vi "GetContainedPathSet.vi"(8 "error in (no error)":errorcluster, 11 "CLabVIEWContainer in":refnum<class "CLabVIEWContainer.lvclass">) -> (0 "error out":errorcluster, 1 "Contained":set{string}(c389), 3 "CLabVIEWContainer out":refnum<class "CLabVIEWContainer.lvclass">)   [LabVIEW 2020, in "LabVIEWContainers.lvlib" / "CLabVIEWContainer.lvclass"]
uses:
  CLabVIEWContainer.lvclass
  CLabVIEWContainer.lvclass/CLabVIEWContainer.ctl
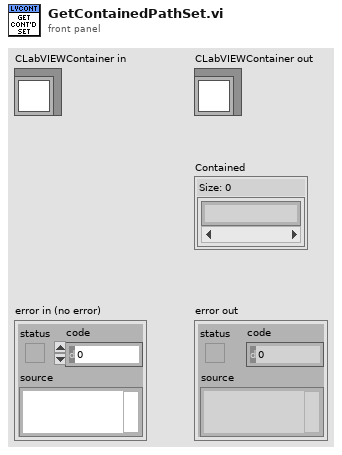
[diagram p1: front panel]
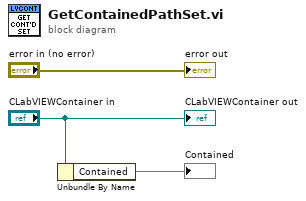
[diagram p0: block diagram]
diagram:
  n1 = Unbundle By Name("CLabVIEWContainer in") -> ("Contained"=→"Contained":set{string})
  "error out" <- "error in (no error)"
  "CLabVIEWContainer out" <- "CLabVIEWContainer in"
